vi "solar_voy Refnum Voyager to SEQ.vi"(1 "Voyager Refnum":T1) -> (0 "Voyager SEQ":refnum<queue>)   [LabVIEW 2018]
doc: "This type casts from the Voyager reference."
uses:
  solar_voy_def/solar_voy_def_ctl PACKET_ID.ctl
  solar_voy_ctl Voyager.ctl
  type/solar_type Item Type.ctl
  solar_voy_def/solar_voy_def_ctl ITEM TYPE.ctl
  solar_voy_def/solar_voy_def_ctl ITEM.ctl
  solar_voy_def/solar_voy_def_ctl PACKET.ctl
  solar_voy_ctl TCP.ctl
  solar_voy_def/solar_voy_def_ctl HDR.ctl
  solar_voy_ctl Port Setup.ctl
  solar_voy_ctl Voyager Refnum.ctl
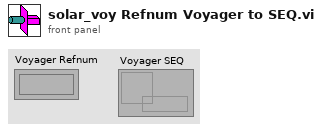
[diagram p1: front panel]
types:
  T1 = typedef "solar_voy_ctl Voyager Refnum.ctl" = refnum<k1>
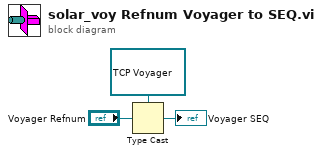
[diagram p0: block diagram]
diagram:
  n1 = Type Cast(type=refnum<queue> refnum ("Voyager SEQ"), x="Voyager Refnum") -> (*(type *) &x=→"Voyager SEQ":refnum<queue>)
